vi "Engine In - Sensor - EGR Cooler Outlet Temp.vi"(10 "Loop Freq (Hz)":sgl, 11 "Raw EGR Cooler Outlet Temp [V]":sgl) -> (3 "EGR Cooler Outlet Temp [C]":sgl)   [LabVIEW 2015, in "ECS-RT.lvlib"]
uses:
  ECS-RT.lvlib
  <vilib>/ptbypt/NI_PtbyPt.lvlib
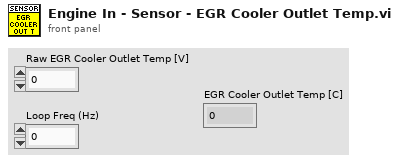
[diagram p1: front panel]
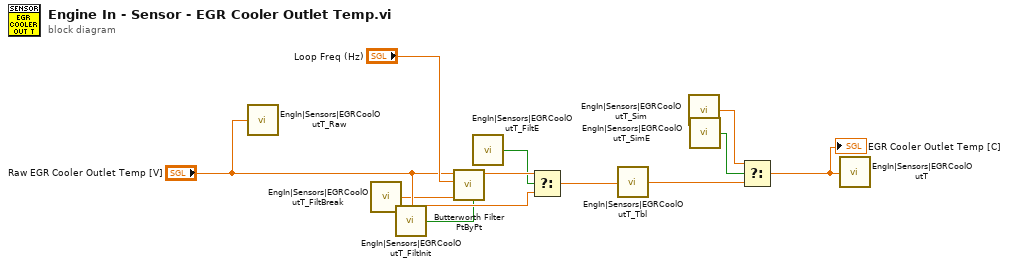
[diagram p0: block diagram]
diagram:
  n1 = call "EngIn|Sensors|EGRCoolOutT_Raw"("Value"="Raw EGR Cooler Outlet Temp [V]") -> ()
  n2 = call "EngIn|Sensors|EGRCoolOutT_FiltBreak"() -> ("Value"=w5:sgl)
  n3 = call "EngIn|Sensors|EGRCoolOutT_FiltInit"() -> ("Value"=w8:bool)
  n4 = call <vilib>:"Butterworth Filter PtByPt.vi"("initialize"=w8, "low cutoff freq: fl"=w5, "sampling freq: fs"="Loop Freq (Hz)", "x"="Raw EGR Cooler Outlet Temp [V]") -> ("Filtered x"=w7:dbl)  [unwired: 5 in, 1 out]
  n5 = call "EngIn|Sensors|EGRCoolOutT_FiltE"() -> ("Value"=w4:bool)
  n6 = Select(t=w7, s=w4, f="Raw EGR Cooler Outlet Temp [V]") -> (s? t:f=w6:dbl)
  n7 = call "EngIn|Sensors|EGRCoolOutT_Tbl"("X Index"=w6) -> ("Y"=w3:sgl)
  n8 = call "EngIn|Sensors|EGRCoolOutT_Sim"() -> ("Value"=w9:sgl)
  n9 = call "EngIn|Sensors|EGRCoolOutT_SimE"() -> ("Value"=w2:bool)
  n10 = Select(t=w9, s=w2, f=w3) -> (s? t:f=w1:sgl)
  "EGR Cooler Outlet Temp [C]" <- w1
  n11 = call "EngIn|Sensors|EGRCoolOutT"("Value"=w1) -> ()
